vi "GetStopUIEvent.vi"(8 "error in (no error)":errorcluster, 11 "Progress in":refnum<class "Progress.lvclass">) -> (0 "error out":errorcluster, 2 "StopUIEvent":refnum<user-event>, 3 "Progress out":refnum<class "Progress.lvclass">)   [LabVIEW 2020, in "Progress.lvlib" / "Progress.lvclass"]
uses:
  Progress.lvclass
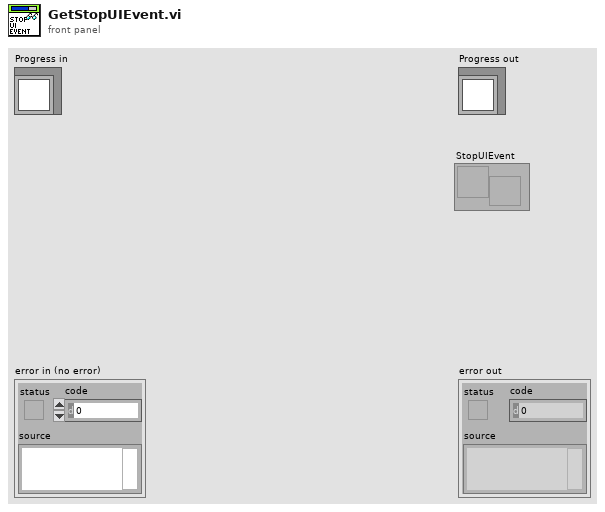
[diagram p1: front panel]
types:
  T1 = typedef "Progress.lvlib/Progress.lvclass/Data.ctl" = cluster{"SlideRefnum":refnum<vi>, "ProgressValue":u64, "NbElement":u64, "Caption":string, "UINotifier":refnum<notifier>, "StopUI":refnum<user-event>}
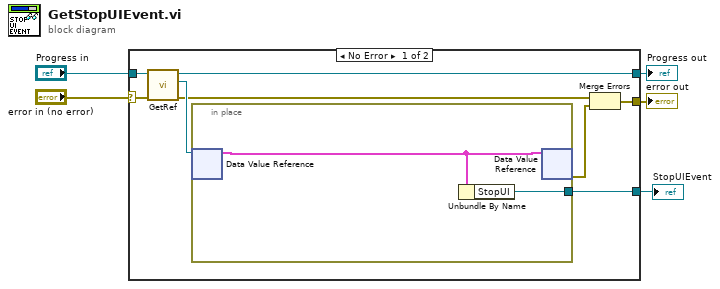
[diagram p0: block diagram]
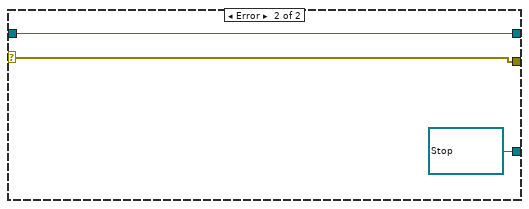
[diagram p2: hidden frame]
diagram:
  n1 = case shown="No Error" "error in (no error)" {
    selector: "error in (no error)" -> [w8 w18]
    tunnel: [w7 w18] -> w4
    tunnel: [w10 w17] -> w2
    tunnel: "Progress in" -> [w9 w17]
    tunnel: [w6 refnum<user-event> refnum ("StopUI")] -> w1
    frame No Error {
      n2 = call "GetRef.vi"("error in (no error)"=w8, "Progress in"=w9) -> ("error out"=w11:errorcluster, "ref"=w13:refnum<data-value>, "Progress out"=w10:refnum<class "Progress.lvclass">)  [unwired: 7 in]
      n3 = in-place {
        in-place-border: [w14] -> w6
        n4 = in-place-dvr #1(w13) -> (w15:T1)  [unwired: 1 out]
        n5 = Unbundle By Name(w15) -> ("StopUI"=w14:refnum<user-event>)
        n6 = in-place-dvr #1(w15) -> (w12:errorcluster)  [unwired: 1 out]
      }
      n7 = Merge Errors(w11, w12) -> (w7:errorcluster)
    }
    frame Error {
    }
  }
  "error out" <- w4
  "Progress out" <- w2
  "StopUIEvent" <- w1
